vi "Example_OE1311&OE1351 Trig in.vi"() -> ()   [LabVIEW 2011]
panel:
  in  "Parameter Index":u16(ring) items=["X", "Y", "R", "θ", "XD1", "YD1", "RD1", "θD1", "XD2", "YD2", "RD2", "θD2", "XD3", "YD3", "RD3", "θD3", "XD4", "YD4", "RD4", "θD4", "XD5", "YD5", "RD5", "θD5", "XD6", "YD6", "RD6", "θD6", "XD7", "YD7", "RD7", "θD7", "X_Noise", "Y_Noise", "Frequency", "AUX-IN1", "AUX-IN2"]
  in  "Trig Mode":u8(ring) items=["Ext_Rissing_Edge", "Ext_Falling_Edge", "Ext_Bilateral_Edge", "Ext_High_Level", "Ext_Low_Level"]
  in  "Trig Source":u8(ring) items=["Internal", "Aux-in1", "Aux-in2"]
  out "Wave":dbl(graph)
  out "loss count":i32=-1
  out "Group":u32
  out "Error out":errorcluster caption="error out"
  in  "function":T1(ring)
  in  "Connect":bool
  in  "Port":u32=10001
  in  "Timeout":u32=100
  in  "IP Address":string="192.168.1.1"
  in  "选项卡控件":enum32{"选项卡 "}(tab)
  in  "Sweep Mode":u16(ring) items=["Linear", "Log"]
  in  "Start Frequency(Hz)":dbl=1000.0 min=1e-05 max=60000000.0 format="%#.3f"
  in  "Stop Frequency(Hz)":dbl=5000.0 min=1e-05 max=60000000.0 format="%#.3f"
  in  "Linear Step Frequency(Hz)":dbl=1000.0 min=1e-05 max=60000000.0 format="%#.3f"
  in  "Log Step Percent(%)":dbl=10.0 min=-100.0 max=100.0 format="%#.2f"
  in  "Step Time(ms)":i32=1000 min=50 max=100000
  in  "Sweep Run Mode":u16(ring) items=["Stop", "Singal", "Loop"]
  in  "Interval Count":u32=1 min=1 max=100000
  in  "Ref_Source":u8(ring) items=["External", "Internal"]
  in  "Sweep":u16(ring) items=["OFF", "ON"]
  out "data_buffer":dbl[][](array[numeric])
  out "cnt":u16
  # "Tel          :   +86-020-84133345\nWebsite  :   www.ssi-instrument.com\nE-mail     :   support@si-instrument.com"
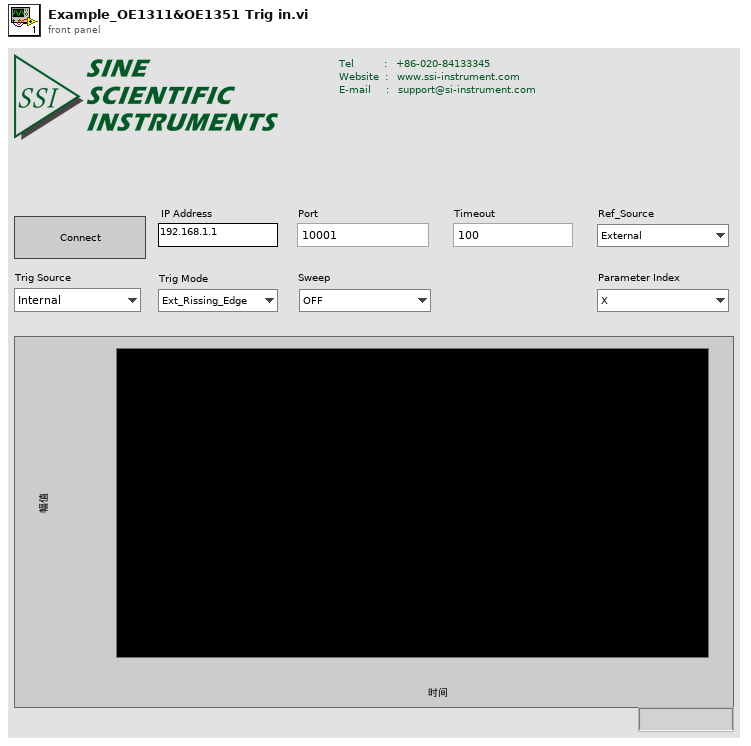
[diagram p1: front panel]
types:
  T1 = enum16{"initial", "Trig In Type", "Sample", "Ext_Sweep_Trig In", "Int_Sweep_Trig In"}
  T2 = enum8{"Enabled", "Disabled", "Disabled and Grayed Out"}
  T3 = cluster{"Port":u32, "Timeout":u32, "IP Address":string}
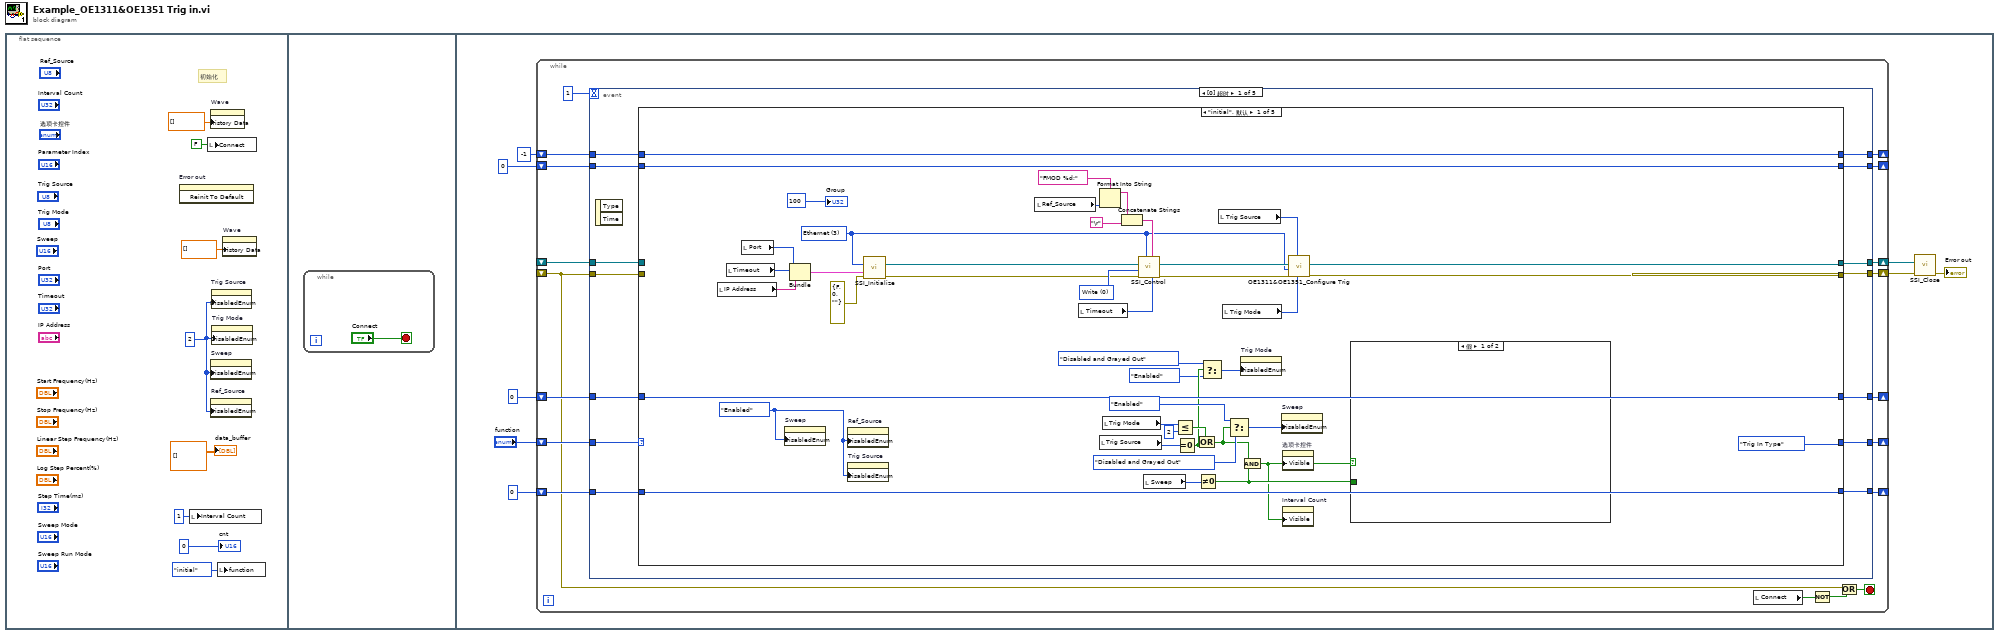
[diagram p0: block diagram]
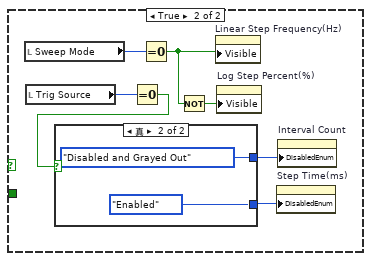
[diagram p2: hidden frame]
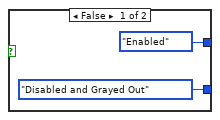
[diagram p3: hidden frame]
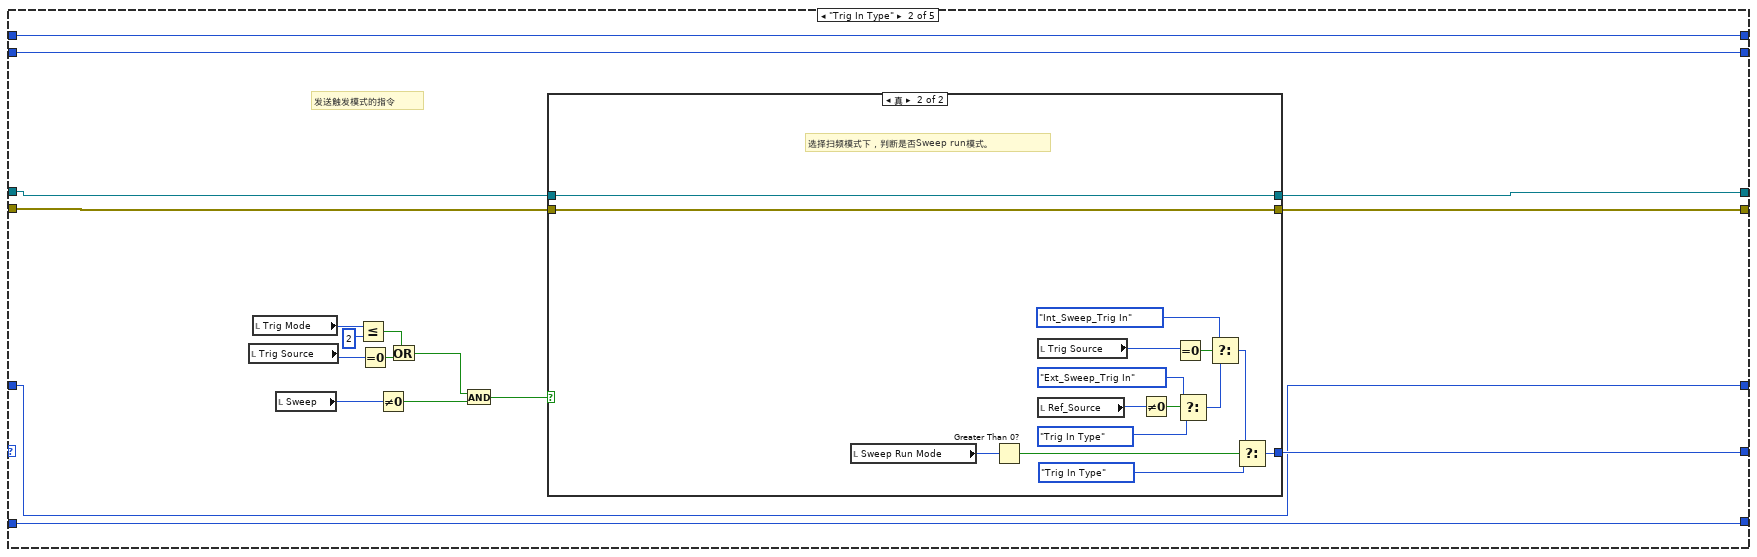
[diagram p4: hidden frame]
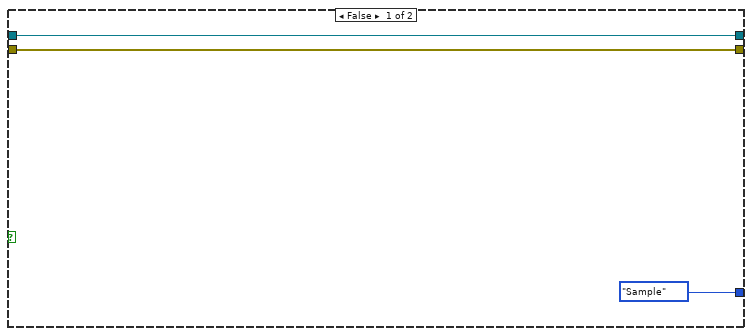
[diagram p5: hidden frame]
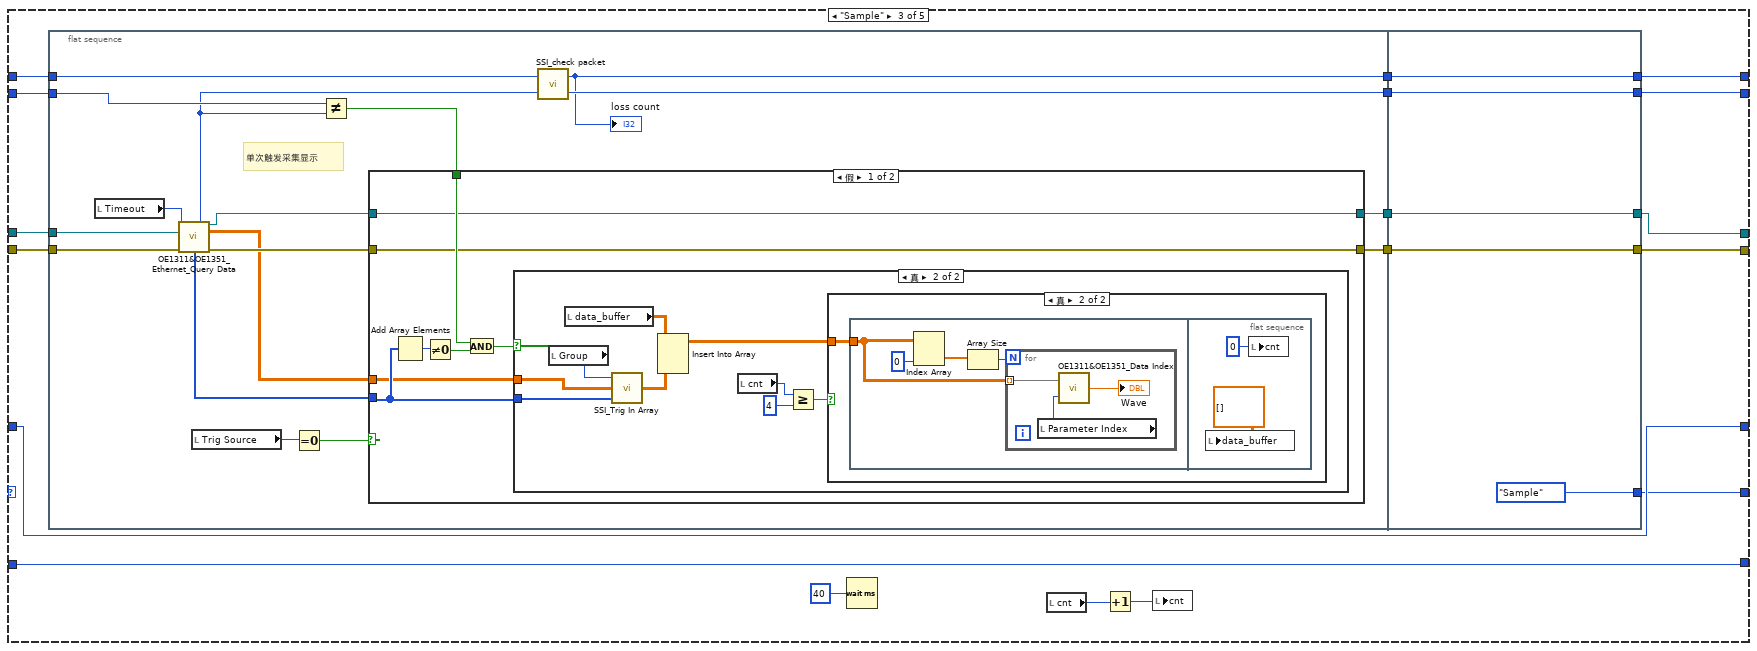
[diagram p6: hidden frame]
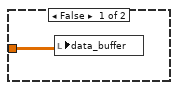
[diagram p8: hidden frame]
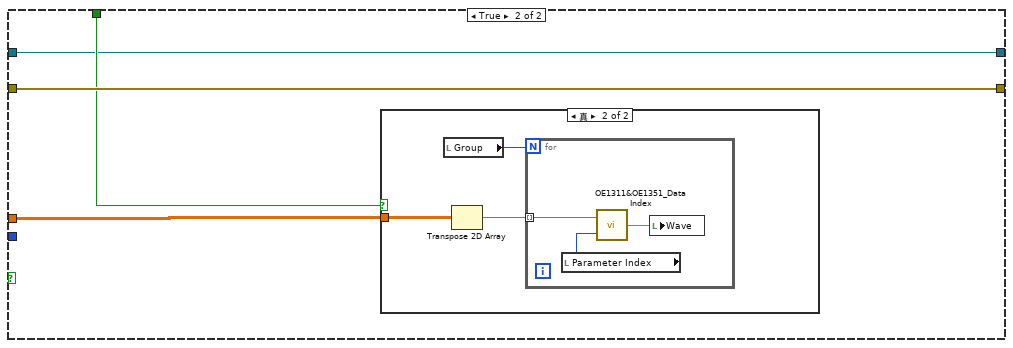
[diagram p9: hidden frame]
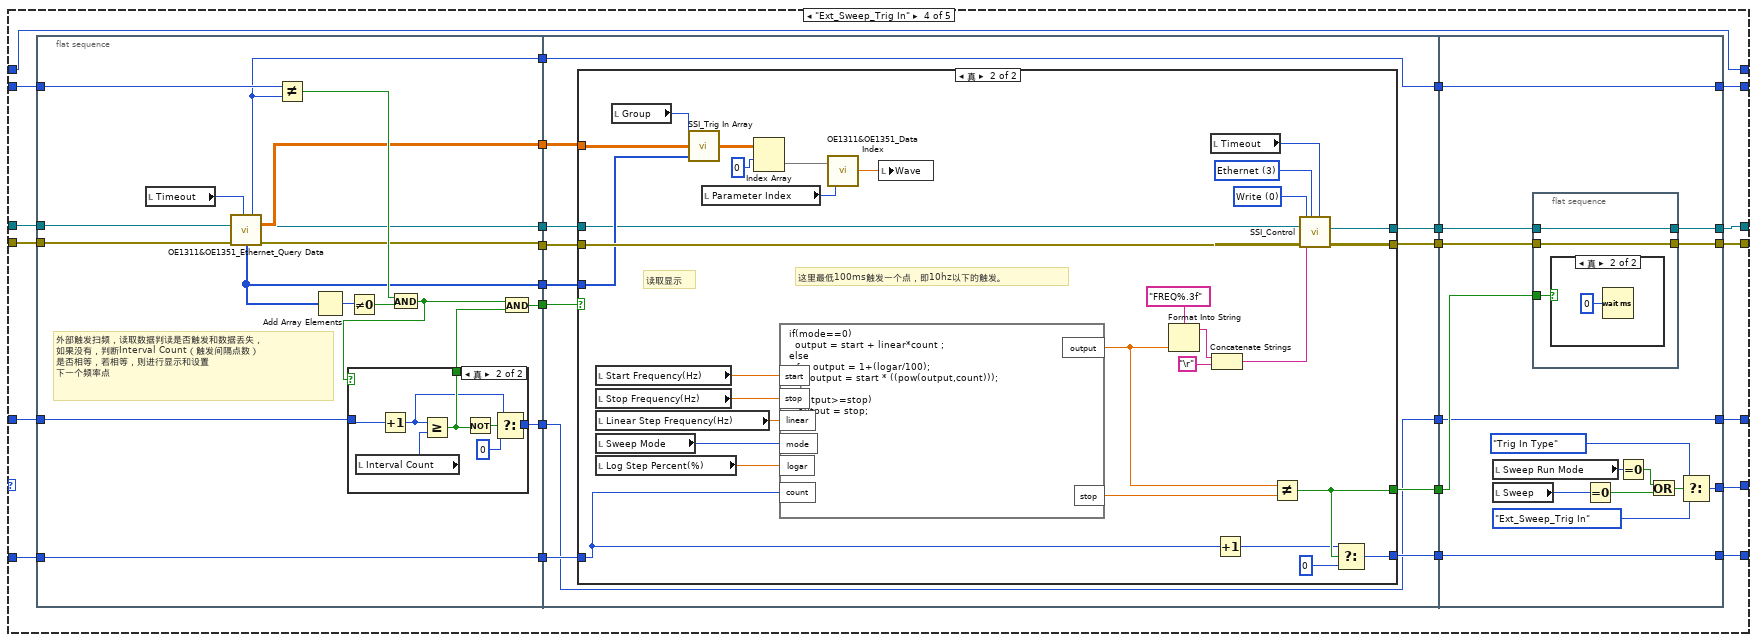
[diagram p11: hidden frame]
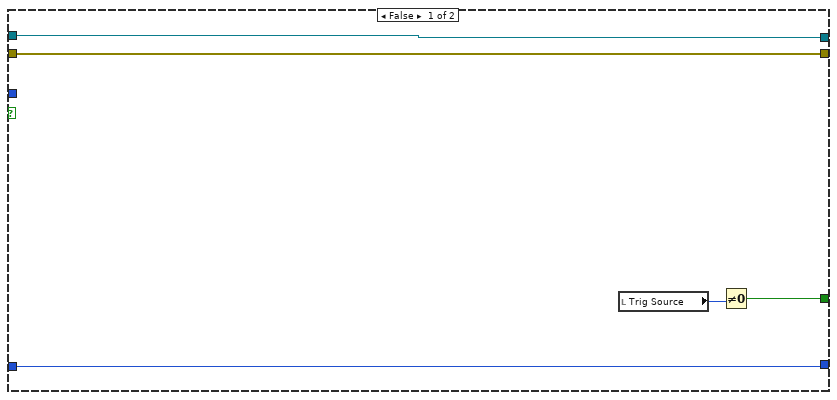
[diagram p13: hidden frame]
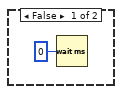
[diagram p14: hidden frame]
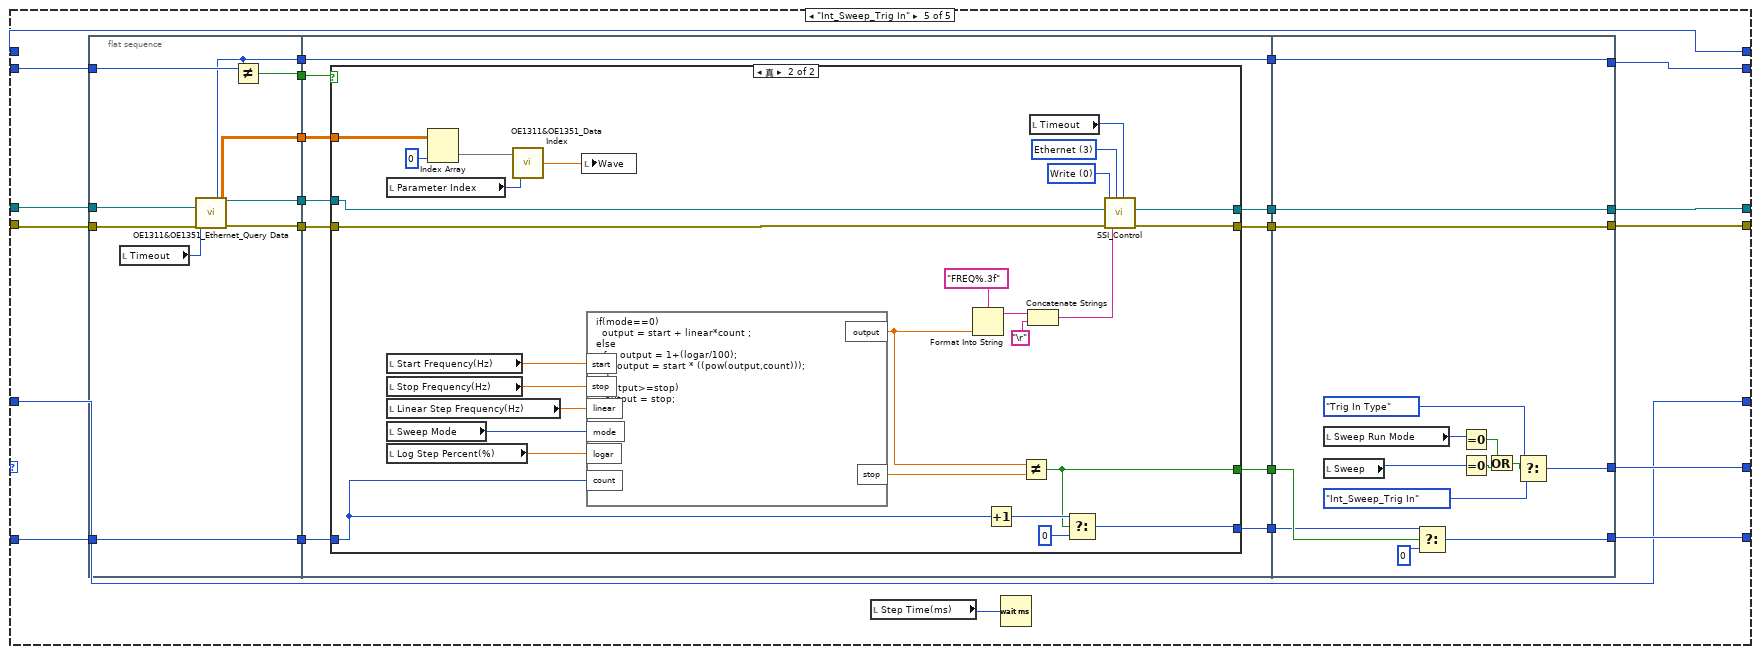
[diagram p15: hidden frame]
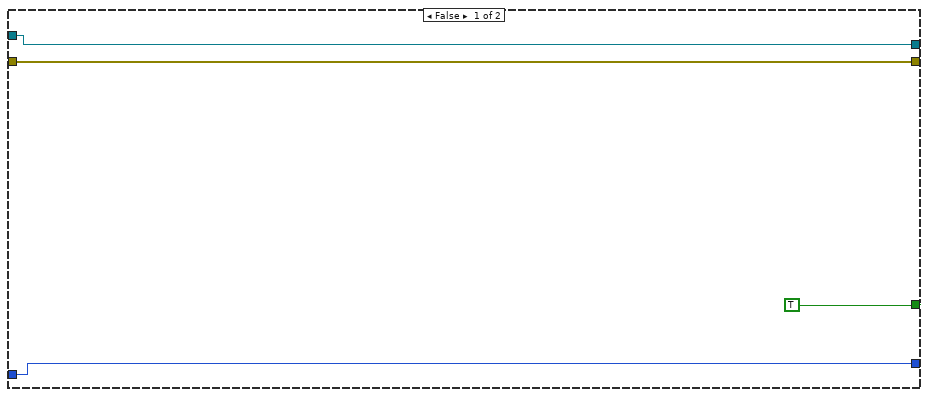
[diagram p16: hidden frame]
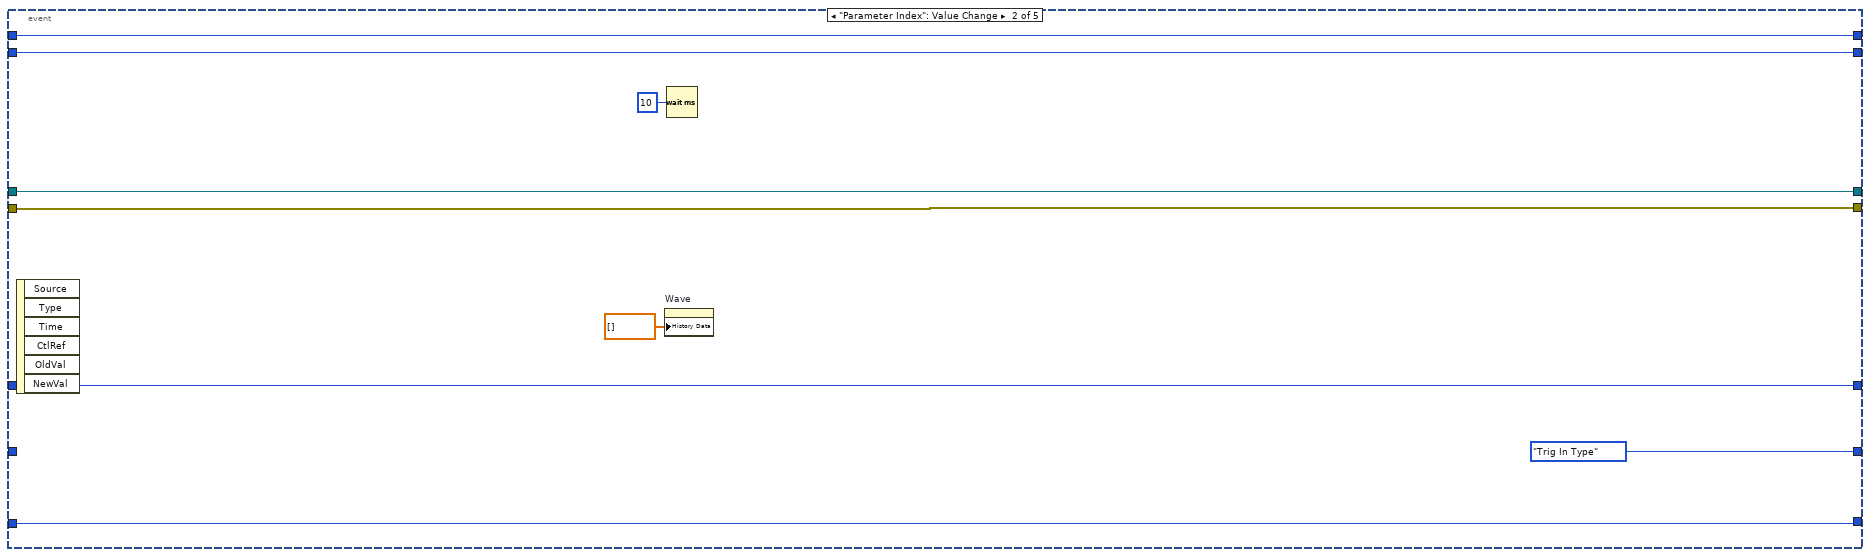
[diagram p17: hidden frame]
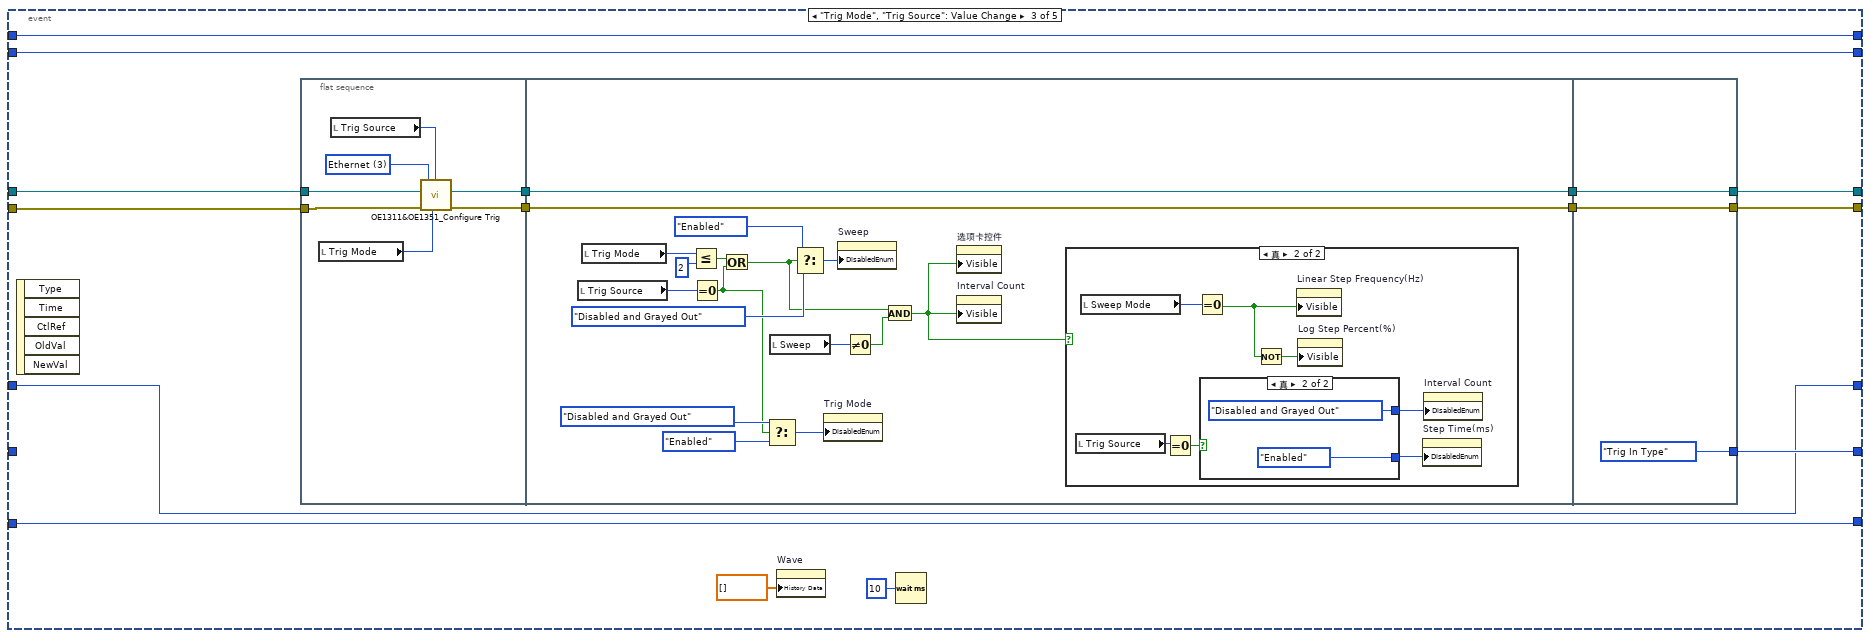
[diagram p18: hidden frame]
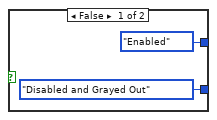
[diagram p20: hidden frame]
diagram:
  n1 = flat-sequence {
    frame #0 {
      w1 = 2
      # "初始化"
      n2 = invoke on="Error out" class="Clust (严格)" method="Reinit To Default"() -> ()  [unwired: 3 in, 3 out]
      n3 = local write "Interval Count"(u32 1 ("Interval Count")) -> ()
      n4 = local write "Connect"(FALSE ("Connect")) -> ()
      n5 = property on="Wave" class="WFChart (严格)"("History Data"=dbl[] [] ("历史数据")) -> ()  [unwired: 2 in, 2 out]
      n6 = property on="Sweep" class="Ring (严格)"("DisabledEnum"=w1) -> ()  [unwired: 2 in, 2 out]
      n7 = property on="Ref_Source" class="Ring (严格)"("DisabledEnum"=w1) -> ()  [unwired: 2 in, 2 out]
      n8 = property on="Trig Source" class="Ring (严格)"("DisabledEnum"=w1) -> ()  [unwired: 2 in, 2 out]
      n9 = property on="Trig Mode" class="Ring (严格)"("DisabledEnum"=w1) -> ()  [unwired: 2 in, 2 out]
      n10 = local write "function"(T1."initial" ("function")) -> ()
      n11 = property on="Wave" class="WFChart (严格)"("History Data"=dbl[] [] ("历史数据")) -> ()  [unwired: 2 in, 2 out]
      "data_buffer" <- dbl[][] []
      "cnt" <- 0
    }
    frame #1 {
      n12 = while {
        stop <- "Connect" stop-if-true
      }
    }
    frame #2 {
      n13 = while {
        shift-right: [w31] -> _
        shift-left: "function" -> [w32]
        shift-right: [w29] -> _
        shift-left: 0 ("f") -> [w30]
        shift-right: [w26] -> _
        shift-left: 0 -> [w27]
        shift-right: [w23] -> _
        shift-left: 0 -> [w24]
        shift-right: [w33] -> w16
        shift-left: _ -> [w22]
        shift-right: [w21] -> w12
        shift-left: _ -> [w20]
        shift-right: [w18] -> _
        shift-left: -1 ("loss count") -> [w19]
        stop <- w34 stop-if-true
        n14 = event shown="[0] 超时" {
          selector: _ -> [_ _ _ _ _]
          dyn-events: _ -> [_ _ _ _ _]
          timeout: 1 -> [_ _ _ _ _]
          tunnel: [w49 w434 w440 w497 w514] -> w33
          tunnel: w22 -> [w48 w434 w444 w498 w514]
          tunnel: w32 -> [w47 _ _ w501 _]
          tunnel: [w46 T1."Trig In Type" ("function") w446 w501 T1."Trig In Type" ("function")] -> w31
          tunnel: w30 -> [w45 w436 w451 w502 w510]
          tunnel: [w44 w436 w451 w502 w510] -> w29
          tunnel: w27 -> [w43 w432 w450 w499 w512]
          tunnel: [w42 w432 w450 w499 w512] -> w26
          tunnel: w24 -> [w41 w431 w445 w500 w509]
          tunnel: [w40 w431 w445 w500 w509] -> w23
          tunnel: [w39 w429 w437 w495 w513] -> w21
          tunnel: w20 -> [w38 w429 w443 w496 w513]
          tunnel: w19 -> [w37 w428 w447 w491 w511]
          tunnel: [w36 w428 w447 w491 w511] -> w18
          event Timeout {
            n15 = event-data() -> ()  [unwired: 1 in, 2 out]
            n16 = case shown="\"initial\", 默认" w47 {
              tunnel: w48 -> [_ w121 w156 w242 w348]
              tunnel: [w81 w120 w149 w240 w358] -> w49
              tunnel: [T1."Trig In Type" ("function") w119 w154 w231 w356] -> w46
              tunnel: w45 -> [w91 w118 w157 w241 w357]
              tunnel: [w91 w118 w157 w239 w355] -> w44
              tunnel: w43 -> [w89 w117 w153 w238 w360]
              tunnel: [w89 w117 w151 w237 w359] -> w42
              tunnel: w41 -> [w90 w116 w155 w225 w354]
              tunnel: [w90 w116 w155 w222 w354] -> w40
              tunnel: [w82 w111 w142 w219 w340] -> w39
              tunnel: w38 -> [_ w112 w144 w221 w344]
              tunnel: w37 -> [w73 w110 w147 w218 w339]
              tunnel: [w73 w110 w141 w218 w339] -> w36
              frame "initial", Default {
                w52 = u16 3 items=["USB", "RS232", "GPIB", "Ethernet"] ("Remote Mode")
                w70 = T2."Enabled" ("禁用")
                w75 = u16 0 items=["Write", "Read"] ("Control")
                n17 = local read "IP Address"() -> (w78:string)
                n18 = local read "Timeout"() -> (w79:u32)
                n19 = local read "Port"() -> (w80:u32)
                n20 = property on="Sweep" class="Ring (严格)"("DisabledEnum"=w70) -> ()  [unwired: 2 in, 2 out]
                n21 = Bundle("Port"=w80, "Timeout"=w79, "IP Address"=w78) -> (w77:T3)  [unwired: 1 in]
                n22 = property on="Ref_Source" class="Ring (严格)"("DisabledEnum"=w70) -> ()  [unwired: 2 in, 2 out]
                n23 = property on="Trig Source" class="Ring (严格)"("DisabledEnum"=w70) -> ()  [unwired: 2 in, 2 out]
                n24 = call "SSI_Initialize.vi"("Remote Mode"=w52, "Ethernet"=w77, "error in (no error)"=errorcluster {"status"=FALSE, "code"=0, "source"=""}) -> ("connection ID(Ethernet)"=w51:refnum<k5>, "error out"=w50:errorcluster)  [unwired: 10 in, 1 out]
                n25 = local read "Ref_Source"() -> (w87:u8)
                n26 = local read "Timeout"() -> (w71:u32)
                n27 = Format Into String(format string="FMOD %d;" ("格式字符串"), w87) -> (resulting string=w88:string)  [unwired: 2 in, 1 out]
                n28 = local read "Trig Source"() -> (w60:u8)
                n29 = local read "Trig Mode"() -> (w58:u8)
                n30 = Concatenate Strings(w88, "\r") -> (w74:string)
                n31 = call "SSI_Control.vi"("Tineout"=w71, "Write Buffer"=w74, "Remote Mode"=w52, "Error in (no error)"=w50, "Control"=w75, "Connection ID in"=w51) -> ("Error out"=w83:errorcluster, "Connection ID out"=w84:refnum<k5>)  [unwired: 2 in, 2 out]
                n32 = local read "Sweep"() -> (w64:u16)
                n33 = Less Or Equal?(x=w58, y=u8 2) -> (x <= y?=w59:bool)
                n34 = Equal To 0?(x=w60) -> (x = 0?=w56:bool)
                n35 = Or(x=w59, y=w56) -> (x .or. y?=w57:bool)
                n36 = Not Equal To 0?(x=w64) -> (x != 0?=w67:bool)
                n37 = Select(t=T2."Disabled and Grayed Out" ("禁用"), s=w56, f=T2."Enabled" ("禁用")) -> (s? t:f=w55:T2)
                n38 = local read "Trig Source"() -> (w68:u8)
                n39 = local read "Trig Mode"() -> (w69:u8)
                n40 = Select(t=T2."Enabled" ("禁用"), s=w57, f=T2."Disabled and Grayed Out") -> (s? t:f=w62:T2)
                n41 = property on="Trig Mode" class="Ring (严格)"("DisabledEnum"=w55) -> ()  [unwired: 2 in, 2 out]
                n42 = And(x=w57, y=w67) -> (x .and. y?=w66:bool)
                n43 = property on="Sweep" class="Ring (严格)"("DisabledEnum"=w62) -> ()  [unwired: 2 in, 2 out]
                n44 = property on="选项卡控件" class="TabCtl (严格)"("Visible"=w66) -> ()  [unwired: 2 in, 2 out]
                n45 = property on="Interval Count" class="DigNum (严格)"("Visible"=w66) -> ()  [unwired: 2 in, 2 out]
                n46 = call "OE1311&OE1351_Configure Trig.vi"("Trig Mode"=w69, "Trig Source"=w68, "Error in (no error)"=w83, "Remote Mode"=w52, "Connection ID in"=w84) -> ("Error out"=w81:errorcluster, "Connection ID out"=w82:refnum<k5>)  [unwired: 3 in, 2 out]
                n47 = case shown="假" w66 {
                  tunnel: w67 -> [_ _]
                  frame False {
                  }
                  frame True {
                    n48 = local read "Sweep Mode"() -> (w98:u16)
                    n49 = local read "Trig Source"() -> (w93:u8)
                    n50 = Equal To 0?(x=w93) -> (x = 0?=w94:bool)
                    n51 = case shown="真" w94 {
                      tunnel: [T2."Disabled and Grayed Out" ("禁用") T2."Enabled" ("禁用")] -> w96
                      tunnel: [T2."Enabled" ("禁用") T2."Disabled and Grayed Out" ("禁用")] -> w95
                      frame False {
                      }
                      frame True {
                      }
                    }
                    n52 = Equal To 0?(x=w98) -> (x = 0?=w99:bool)
                    n53 = Not(x=w99) -> (.not. x?=w97:bool)
                    n54 = property on="Linear Step Frequency(Hz)" class="DigNum (严格)"("Visible"=w99) -> ()  [unwired: 2 in, 2 out]
                    n55 = property on="Log Step Percent(%)" class="DigNum (严格)"("Visible"=w97) -> ()  [unwired: 2 in, 2 out]
                    n56 = property on="Step Time(ms)" class="DigNum (严格)"("DisabledEnum"=w96) -> ()  [unwired: 2 in, 2 out]
                    n57 = property on="Interval Count" class="DigNum (严格)"("DisabledEnum"=w95) -> ()  [unwired: 2 in, 2 out]
                  }
                }
                "Group" <- 100
              }
              frame "Trig In Type" {
                # "发送触发模式的指令"
                n58 = local read "Trig Source"() -> (w106:u8)
                n59 = local read "Trig Mode"() -> (w109:u8)
                n60 = local read "Sweep"() -> (w114:u16)
                n61 = Less Or Equal?(x=w109, y=u8 2) -> (x <= y?=w107:bool)
                n62 = Equal To 0?(x=w106) -> (x = 0?=w108:bool)
                n63 = Not Equal To 0?(x=w114) -> (x != 0?=w113:bool)
                n64 = Or(x=w107, y=w108) -> (x .or. y?=w104:bool)
                n65 = And(x=w104, y=w113) -> (x .and. y?=w115:bool)
                n66 = case shown="真" w115 {
                  tunnel: [w124 w135] -> w120
                  tunnel: w121 -> [w124 w135]
                  tunnel: [T1."Sample" ("function") w138] -> w119
                  tunnel: w112 -> [w122 w126]
                  tunnel: [w122 w126] -> w111
                  frame False {
                  }
                  frame True {
                    # "选择扫频模式下，判断是否Sweep run模式。"
                    n67 = local read "Sweep Run Mode"() -> (w136:u16)
                    n68 = Greater Than 0?(x=w136) -> (x > 0?=w139:bool)
                    n69 = local read "Trig Source"() -> (w125:u8)
                    n70 = local read "Ref_Source"() -> (w134:u8)
                    n71 = Not Equal To 0?(x=w134) -> (x != 0?=w133:bool)
                    n72 = Equal To 0?(x=w125) -> (x = 0?=w131:bool)
                    n73 = Select(t=T1."Ext_Sweep_Trig In" ("function"), s=w133, f=T1."Trig In Type" ("function")) -> (s? t:f=w132:T1)
                    n74 = Select(t=T1."Int_Sweep_Trig In" ("function"), s=w131, f=w132) -> (s? t:f=w137:T1)
                    n75 = Select(t=w137, s=w139, f=T1."Trig In Type" ("function")) -> (s? t:f=w138:T1)
                  }
                }
              }
              frame "Sample" {
                n76 = flat-sequence {
                  tunnel: w156 -> [w173]
                  tunnel: w153 -> [w170]
                  tunnel: [w167] -> w152
                  tunnel: [w168] -> w150
                  tunnel: w147 -> [w166]
                  tunnel: w144 -> [w164]
                  tunnel: [w162] -> w143
                  tunnel: [w161] -> w140
                  tunnel: w152 -> [w216]
                  tunnel: w150 -> [w215]
                  tunnel: [T1."Sample" ("function")] -> w154
                  tunnel: [w216] -> w151
                  tunnel: [w215] -> w149
                  tunnel: w143 -> [w213]
                  tunnel: [w213] -> w142
                  tunnel: [w212] -> w141
                  tunnel: w140 -> [w212]
                  frame #0 {
                    # "单次触发采集显示"
                    n77 = local read "Timeout"() -> (w160:u32)
                    n78 = call "OE1311&OE1351_Ethernet_Query Data.vi"("Connection ID in"=w164, "Timeout"=w160, "Error in (no error)"=w173) -> ("Buffer Count"=w167:u8, "Connection ID out"=w163:refnum<k5>, "Total Date Array"=w165:dbl[][], "Trig_Count"=w171:u8[], "Error out"=w169:errorcluster)  [unwired: 5 in, 3 out]
                    n79 = local read "Trig Source"() -> (w159:u8)
                    n80 = Equal To 0?(x=w159) -> (x = 0?=w172:bool)
                    n81 = Not Equal?(x=w170, y=w167) -> (x != y?=w158:bool)
                    n82 = case shown="假" w172 {
                      tunnel: w165 -> [w177 w204]
                      tunnel: w171 -> [w180 _]
                      tunnel: w158 -> [w176 w203]
                      tunnel: w169 -> [w174 w205]
                      tunnel: [w174 w205] -> w168
                      tunnel: w163 -> [w175 w202]
                      tunnel: [w175 w202] -> w162
                      frame False {
                        n83 = Add Array Elements(numeric array=w180) -> (sum=w181:u8)
                        n84 = Not Equal To 0?(x=w181) -> (x != 0?=w179:bool)
                        n85 = And(x=w176, y=w179) -> (x .and. y?=w178:bool)
                        n86 = case shown="真" w178 {
                          tunnel: w177 -> [_ w190]
                          tunnel: w180 -> [_ w189]
                          frame False {
                          }
                          frame True {
                            n87 = local read "Group"() -> (w188:u32)
                            n88 = local read "data_buffer"() -> (w187:dbl[][])
                            n89 = call "SSI_Trig In Array.vi"("Trig_Count"=w189, "Input Array"=w190, "Group"=w188) -> ("Output Array"=w186:dbl[][])
                            n90 = Insert Into Array(array=w187, new element=w186) -> (w185:dbl[][])  [unwired: 2 in]
                            n91 = local read "cnt"() -> (w184:u16)
                            n92 = Greater Or Equal?(x=w184, y=u16 4) -> (x >= y?=w182:bool)
                            n93 = case shown="真" w182 {
                              tunnel: w185 -> [w191 w192]
                              frame False {
                                n94 = local write "data_buffer"(w191) -> ()
                              }
                              frame True {
                                n95 = flat-sequence {
                                tunnel: w192 -> [w194]
                                frame #0 {
                                n96 = Index Array(array=w194, index (col)=0 ("禁用的索引 (列)")) -> (element=w193:dbl[])  [unwired: 1 in]
                                n97 = Array Size(array=w193) -> (size(s)=w196:i32)
                                n98 = for {
                                N: w196 -> [_]
                                tunnel: w194 -> [w198] mode=indexing
                                n99 = local read "Parameter Index"() -> (w197:u16)
                                n100 = call "OE1311&OE1351_Data Index.vi"("Parameter Type"=w197, "Input Date Array"=w198) -> ("Parameter"=→"Wave":dbl)
                                }
                                }
                                frame #1 {
                                n101 = local write "data_buffer"(dbl[][] [] ("data_buffer")) -> ()
                                n102 = local write "cnt"(u16 0 ("cnt")) -> ()
                                }
                                }
                              }
                            }
                          }
                        }
                      }
                      frame True {
                        n103 = case shown="真" w203 {
                          tunnel: w204 -> [_ w208]
                          frame False {
                          }
                          frame True {
                            n104 = local read "Group"() -> (w207:u32)
                            n105 = Transpose 2D Array(2D array=w208) -> (transposed array=w206:dbl[][])
                            n106 = for {
                              N: w207 -> [_]
                              tunnel: w206 -> [w211] mode=indexing
                              n107 = local read "Parameter Index"() -> (w209:u16)
                              n108 = call "OE1311&OE1351_Data Index.vi"("Parameter Type"=w209, "Input Date Array"=w211) -> ("Parameter"=w210:dbl)
                              n109 = local write "Wave"(w210) -> ()
                            }
                          }
                        }
                      }
                    }
                    n110 = call "SSI_check packet.vi"("input"=w167, "input loss"=w166) -> ("loss count"=w161:i32)  [unwired: 1 out]
                    "loss count" <- w161
                  }
                  frame #1 {
                  }
                }
                n111 = Wait (ms)(milliseconds to wait=40) -> ()  [unwired: 1 out]
                n112 = local read "cnt"() -> (w145:u16)
                n113 = Increment(x=w145) -> (x+1=w146:u16)
                n114 = local write "cnt"(w146) -> ()
              }
              frame "Ext_Sweep_Trig In" {
                n115 = flat-sequence {
                  tunnel: w242 -> [w259]
                  tunnel: w241 -> [w257]
                  tunnel: w238 -> [w260]
                  tunnel: [w257] -> w236
                  tunnel: [w258] -> w235
                  tunnel: [w253] -> w229
                  tunnel: [w252] -> w228
                  tunnel: [w251] -> w227
                  tunnel: [w250] -> w226
                  tunnel: w225 -> [w248]
                  tunnel: [w246] -> w224
                  tunnel: w221 -> [w245]
                  tunnel: [w244] -> w217
                  tunnel: w235 -> [w271]
                  tunnel: w236 -> [w278]
                  tunnel: [w279] -> w234
                  tunnel: [w277] -> w233
                  tunnel: [w271] -> w232
                  tunnel: [w276] -> w230
                  tunnel: w229 -> [w280]
                  tunnel: w228 -> [w275]
                  tunnel: w227 -> [w274]
                  tunnel: w226 -> [w273]
                  tunnel: w224 -> [w272]
                  tunnel: [w272] -> w223
                  tunnel: [w270] -> w220
                  tunnel: w217 -> [w269]
                  tunnel: [w331] -> w237
                  tunnel: [w332] -> w239
                  tunnel: [w329] -> w240
                  tunnel: w234 -> [w330]
                  tunnel: w233 -> [w332]
                  tunnel: w232 -> [w331]
                  tunnel: [w326] -> w231
                  tunnel: w230 -> [w328]
                  tunnel: w223 -> [w327]
                  tunnel: [w327] -> w222
                  tunnel: w220 -> [w322]
                  tunnel: [w321] -> w219
                  frame #0 {
                    # "外部触发扫频，读取数据判读是否触发和数据丢失，\n如果没有，判断Interval Count（触发间隔点数）\n是否相等，若相等，则进行显示和设置\n下一个频率点"
                    n116 = local read "Timeout"() -> (w243:u32)
                    n117 = call "OE1311&OE1351_Ethernet_Query Data.vi"("Connection ID in"=w245, "Timeout"=w243, "Error in (no error)"=w259) -> ("Buffer Count"=w258:u8, "Connection ID out"=w244:refnum<k5>, "Total Date Array"=w252:dbl[][], "Trig_Count"=w251:u8[], "Error out"=w253:errorcluster)  [unwired: 5 in, 3 out]
                    n118 = Not Equal?(x=w260, y=w258) -> (x != y?=w255:bool)
                    n119 = Add Array Elements(numeric array=w251) -> (sum=w256:u8)
                    n120 = Not Equal To 0?(x=w256) -> (x != 0?=w254:bool)
                    n121 = And(x=w255, y=w254) -> (x .and. y?=w249:bool)
                    n122 = case shown="真" w249 {
                      tunnel: w248 -> [w261 w268]
                      tunnel: [_ w265] -> w247
                      tunnel: [w261 w262] -> w246
                      frame False {
                      }
                      frame True {
                        n123 = local read "Interval Count"() -> (w267:u32)
                        n124 = Increment(x=w268) -> (x+1=w264:i32)
                        n125 = Greater Or Equal?(x=w264, y=w267) -> (x >= y?=w265:bool)
                        n126 = Not(x=w265) -> (.not. x?=w266:bool)
                        n127 = Select(t=w264, s=w266, f=0) -> (s? t:f=w262:i32)
                      }
                    }
                    n128 = And(x=w249, y=w247) -> (x .and. y?=w250:bool)
                  }
                  frame #1 {
                    n129 = case shown="真" w273 {
                      tunnel: w280 -> [w285 w299]
                      tunnel: [w285 w301] -> w279
                      tunnel: w278 -> [w284 w307]
                      tunnel: [w284 w306] -> w277
                      tunnel: [w283 w305] -> w276
                      tunnel: w275 -> [_ w298]
                      tunnel: w274 -> [_ w296]
                      tunnel: w269 -> [w282 w293]
                      tunnel: [w282 w292] -> w270
                      frame False {
                        n130 = local read "Trig Source"() -> (w281:u8)
                        n131 = Not Equal To 0?(x=w281) -> (x != 0?=w283:bool)
                      }
                      frame True {
                        w289 = u16 3 items=["USB", "RS232", "GPIB", "Ethernet"] ("Remote Mode")
                        w291 = u16 0 items=["Write", "Read"] ("Control")
                        # "这里最低100ms触发一个点，即10hz以下的触发。"
                        # "读取显示"
                        n132 = local read "Start Frequency(Hz)"() -> (w313:dbl)
                        n133 = local read "Stop Frequency(Hz)"() -> (w312:dbl)
                        n134 = local read "Linear Step Frequency(Hz)"() -> (w311:dbl)
                        n135 = local read "Sweep Mode"() -> (w310:u16)
                        n136 = local read "Log Step Percent(%)"() -> (w309:dbl)
                        n137 = local read "Group"() -> (w297:u32)
                        n138 = call "SSI_Trig In Array.vi"("Trig_Count"=w296, "Input Array"=w298, "Group"=w297) -> ("Output Array"=w295:dbl[][])
                        n139 = local read "Parameter Index"() -> (w288:u16)
                        n140 = Index Array(array=w295, index (row)=0 ("索引 (行)")) -> (element=w294:dbl[])  [unwired: 1 in]
                        n141 = formula code="if(mode==0)\n  output = start + linear*count ;\nelse \n  {    output = 1+(logar/100);\n       output = start * ((pow(output,count)));\n   }\nif(output>=stop)\n   output = stop;"("start"=w313, "stop"=w312, "linear"=w311, "logar"=w309, "mode"=w310, "count"=w307) -> ("stop"=w308:dbl, "output"=w302:dbl)
                        n142 = call "OE1311&OE1351_Data Index.vi"("Parameter Type"=w288, "Input Date Array"=w294) -> ("Parameter"=w287:dbl)
                        n143 = local write "Wave"(w287) -> ()
                        n144 = Format Into String(format string="FREQ%.3f" ("格式字符串"), w302) -> (resulting string=w315:string)  [unwired: 2 in, 1 out]
                        n145 = local read "Timeout"() -> (w290:u32)
                        n146 = Concatenate Strings(w315, "\r") -> (w300:string)
                        n147 = Increment(x=w307) -> (x+1=w304:i32)
                        n148 = Not Equal?(x=w302, y=w308) -> (x != y?=w305:bool)
                        n149 = call "SSI_Control.vi"("Tineout"=w290, "Write Buffer"=w300, "Remote Mode"=w289, "Error in (no error)"=w299, "Control"=w291, "Connection ID in"=w293) -> ("Error out"=w301:errorcluster, "Connection ID out"=w292:refnum<k5>)  [unwired: 2 in, 2 out]
                        n150 = Select(t=w304, s=w305, f=0) -> (s? t:f=w306:i32)
                      }
                    }
                  }
                  frame #2 {
                    n151 = local read "Sweep Run Mode"() -> (w317:u16)
                    n152 = local read "Sweep"() -> (w325:u16)
                    n153 = flat-sequence {
                      tunnel: [w335] -> w329
                      tunnel: w330 -> [w335]
                      tunnel: w328 -> [w334]
                      tunnel: [w333] -> w321
                      tunnel: w322 -> [w333]
                      frame #0 {
                        n154 = case shown="真" w334 {
                          frame False {
                            n155 = Wait (ms)(milliseconds to wait=u32 0 ("等待时间（毫秒）")) -> ()  [unwired: 1 out]
                          }
                          frame True {
                            n156 = Wait (ms)(milliseconds to wait=u32 0 ("等待时间（毫秒）")) -> ()  [unwired: 1 out]
                          }
                        }
                      }
                    }
                    n157 = Equal To 0?(x=w325) -> (x = 0?=w319:bool)
                    n158 = Equal To 0?(x=w317) -> (x = 0?=w318:bool)
                    n159 = Or(x=w318, y=w319) -> (x .or. y?=w320:bool)
                    n160 = Select(t=T1."Trig In Type" ("function"), s=w320, f=T1."Ext_Sweep_Trig In" ("function")) -> (s? t:f=w326:T1)
                  }
                }
              }
              frame "Int_Sweep_Trig In" {
                n161 = flat-sequence {
                  tunnel: [w367] -> w353
                  tunnel: [w366] -> w351
                  tunnel: w360 -> [w370]
                  tunnel: w357 -> [w368]
                  tunnel: w348 -> [w365]
                  tunnel: [w369] -> w347
                  tunnel: [w368] -> w346
                  tunnel: w344 -> [w364]
                  tunnel: [w363] -> w343
                  tunnel: [w362] -> w342
                  tunnel: w353 -> [w380]
                  tunnel: [w380] -> w352
                  tunnel: w351 -> [w379]
                  tunnel: [w378] -> w350
                  tunnel: [w374] -> w349
                  tunnel: w347 -> [w377]
                  tunnel: w346 -> [w376]
                  tunnel: [w375] -> w345
                  tunnel: w343 -> [w373]
                  tunnel: w342 -> [w372]
                  tunnel: [w371] -> w341
                  tunnel: [w427] -> w359
                  tunnel: w352 -> [w427]
                  tunnel: [w426] -> w358
                  tunnel: w350 -> [w426]
                  tunnel: [w420] -> w356
                  tunnel: [w425] -> w355
                  tunnel: w349 -> [w423]
                  tunnel: w345 -> [w422]
                  tunnel: w341 -> [w417]
                  tunnel: [w417] -> w340
                  frame #0 {
                    n162 = local read "Timeout"() -> (w361:u32)
                    n163 = call "OE1311&OE1351_Ethernet_Query Data.vi"("Connection ID in"=w364, "Timeout"=w361, "Error in (no error)"=w365) -> ("Buffer Count"=w367:u8, "Connection ID out"=w362:refnum<k5>, "Total Date Array"=w363:dbl[][], "Error out"=w366:errorcluster)  [unwired: 5 in, 4 out]
                    n164 = Not Equal?(x=w370, y=w367) -> (x != y?=w369:bool)
                  }
                  frame #1 {
                    n165 = case shown="真" w377 {
                      tunnel: [w384 w394] -> w378
                      tunnel: w379 -> [w384 w395]
                      tunnel: w376 -> [w383 w406]
                      tunnel: [w383 w400] -> w375
                      tunnel: [TRUE w401] -> w374
                      tunnel: w373 -> [_ w392]
                      tunnel: w372 -> [w381 w391]
                      tunnel: [w381 w389] -> w371
                      frame False {
                      }
                      frame True {
                        w387 = u16 3 items=["USB", "RS232", "GPIB", "Ethernet"] ("Remote Mode")
                        w390 = u16 0 items=["Write", "Read"] ("Control")
                        n166 = local read "Parameter Index"() -> (w386:u16)
                        n167 = local read "Start Frequency(Hz)"() -> (w412:dbl)
                        n168 = local read "Stop Frequency(Hz)"() -> (w411:dbl)
                        n169 = local read "Linear Step Frequency(Hz)"() -> (w410:dbl)
                        n170 = local read "Sweep Mode"() -> (w409:u16)
                        n171 = local read "Log Step Percent(%)"() -> (w408:dbl)
                        n172 = Index Array(array=w392, index (col)=0 ("禁用的索引 (列)")) -> (element=w396:dbl[])  [unwired: 1 in]
                        n173 = call "OE1311&OE1351_Data Index.vi"("Parameter Type"=w386, "Input Date Array"=w396) -> ("Parameter"=w385:dbl)
                        n174 = local write "Wave"(w385) -> ()
                        n175 = formula code="if(mode==0)\n  output = start + linear*count ;\nelse \n  {    output = 1+(logar/100);\n       output = start * ((pow(output,count)));\n   }\nif(output>=stop)\n   output = stop;"("start"=w412, "stop"=w411, "linear"=w410, "logar"=w408, "mode"=w409, "count"=w406) -> ("stop"=w402:dbl, "output"=w398:dbl)
                        n176 = Format Into String(format string="FREQ%.3f" ("格式字符串"), w398) -> (resulting string=w403:string)  [unwired: 2 in, 1 out]
                        n177 = Increment(x=w406) -> (x+1=w407:i32)
                        n178 = Not Equal?(x=w398, y=w402) -> (x != y?=w401:bool)
                        n179 = Concatenate Strings(w403, "\r") -> (w393:string)
                        n180 = local read "Timeout"() -> (w388:u32)
                        n181 = Select(t=w407, s=w401, f=0) -> (s? t:f=w400:i32)
                        n182 = call "SSI_Control.vi"("Tineout"=w388, "Write Buffer"=w393, "Remote Mode"=w387, "Error in (no error)"=w395, "Control"=w390, "Connection ID in"=w391) -> ("Error out"=w394:errorcluster, "Connection ID out"=w389:refnum<k5>)  [unwired: 2 in, 2 out]
                      }
                    }
                  }
                  frame #2 {
                    n183 = local read "Sweep Run Mode"() -> (w413:u16)
                    n184 = local read "Sweep"() -> (w421:u16)
                    n185 = Select(t=w422, s=w423, f=u16 0) -> (s? t:f=w425:i32)
                    n186 = Equal To 0?(x=w413) -> (x = 0?=w414:bool)
                    n187 = Equal To 0?(x=w421) -> (x = 0?=w415:bool)
                    n188 = Or(x=w414, y=w415) -> (x .or. y?=w416:bool)
                    n189 = Select(t=T1."Trig In Type" ("function"), s=w416, f=T1."Int_Sweep_Trig In" ("function")) -> (s? t:f=w420:T1)
                  }
                }
                n190 = local read "Step Time(ms)"() -> (w338:i32)
                n191 = Wait (ms)(milliseconds to wait=w338) -> ()  [unwired: 1 out]
              }
            }
          }
          event "Parameter Index": Value Change {
            n192 = event-data() -> ()  [unwired: 1 in, 6 out]
            n193 = property on="Wave" class="WFChart (严格)"("History Data"=dbl[] [] ("历史数据")) -> ()  [unwired: 2 in, 2 out]
            n194 = Wait (ms)(milliseconds to wait=u32 10 ("等待时间（毫秒）")) -> ()  [unwired: 1 out]
          }
          event "Trig Mode", "Trig Source": Value Change {
            n195 = event-data() -> ()  [unwired: 1 in, 5 out]
            n196 = flat-sequence {
              tunnel: w444 -> [w457]
              tunnel: w443 -> [w458]
              tunnel: [w455] -> w441
              tunnel: [w454] -> w438
              tunnel: [w468] -> w442
              tunnel: w441 -> [w468]
              tunnel: [w467] -> w439
              tunnel: w438 -> [w467]
              tunnel: [T1."Trig In Type" ("function")] -> w446
              tunnel: w442 -> [w488]
              tunnel: [w488] -> w440
              tunnel: w439 -> [w487]
              tunnel: [w487] -> w437
              frame #0 {
                w456 = u16 3 items=["USB"=0, "Ethernet"=3] ("Remote Mode")
                n197 = local read "Trig Mode"() -> (w453:u8)
                n198 = local read "Trig Source"() -> (w452:u8)
                n199 = call "OE1311&OE1351_Configure Trig.vi"("Trig Mode"=w453, "Trig Source"=w452, "Error in (no error)"=w457, "Remote Mode"=w456, "Connection ID in"=w458) -> ("Error out"=w455:errorcluster, "Connection ID out"=w454:refnum<k5>)  [unwired: 3 in, 2 out]
              }
              frame #1 {
                n200 = local read "Trig Source"() -> (w464:u8)
                n201 = local read "Trig Mode"() -> (w463:u8)
                n202 = Less Or Equal?(x=w463, y=u8 2) -> (x <= y?=w466:bool)
                n203 = Equal To 0?(x=w464) -> (x = 0?=w459:bool)
                n204 = Or(x=w466, y=w459) -> (x .or. y?=w465:bool)
                n205 = Select(t=T2."Disabled and Grayed Out" ("禁用"), s=w459, f=T2."Enabled" ("禁用")) -> (s? t:f=w462:T2)
                n206 = local read "Sweep"() -> (w470:u16)
                n207 = Select(t=T2."Enabled" ("禁用"), s=w465, f=T2."Disabled and Grayed Out") -> (s? t:f=w474:T2)
                n208 = property on="Trig Mode" class="Ring (严格)"("DisabledEnum"=w462) -> ()  [unwired: 2 in, 2 out]
                n209 = property on="Sweep" class="Ring (严格)"("DisabledEnum"=w474) -> ()  [unwired: 2 in, 2 out]
                n210 = Not Equal To 0?(x=w470) -> (x != 0?=w469:bool)
                n211 = And(x=w465, y=w469) -> (x .and. y?=w471:bool)
                n212 = property on="选项卡控件" class="TabCtl (严格)"("Visible"=w471) -> ()  [unwired: 2 in, 2 out]
                n213 = property on="Interval Count" class="DigNum (严格)"("Visible"=w471) -> ()  [unwired: 2 in, 2 out]
                n214 = case shown="真" w471 {
                  frame False {
                  }
                  frame True {
                    n215 = local read "Trig Source"() -> (w476:u8)
                    n216 = local read "Sweep Mode"() -> (w481:u16)
                    n217 = Equal To 0?(x=w476) -> (x = 0?=w477:bool)
                    n218 = Equal To 0?(x=w481) -> (x = 0?=w482:bool)
                    n219 = case shown="真" w477 {
                      tunnel: [T2."Disabled and Grayed Out" ("禁用") T2."Enabled" ("禁用")] -> w479
                      tunnel: [T2."Enabled" ("禁用") T2."Disabled and Grayed Out" ("禁用")] -> w478
                      frame False {
                      }
                      frame True {
                      }
                    }
                    n220 = Not(x=w482) -> (.not. x?=w480:bool)
                    n221 = property on="Linear Step Frequency(Hz)" class="DigNum (严格)"("Visible"=w482) -> ()  [unwired: 2 in, 2 out]
                    n222 = property on="Log Step Percent(%)" class="DigNum (严格)"("Visible"=w480) -> ()  [unwired: 2 in, 2 out]
                    n223 = property on="Step Time(ms)" class="DigNum (严格)"("DisabledEnum"=w479) -> ()  [unwired: 2 in, 2 out]
                    n224 = property on="Interval Count" class="DigNum (严格)"("DisabledEnum"=w478) -> ()  [unwired: 2 in, 2 out]
                  }
                }
              }
              frame #2 {
              }
            }
            n225 = property on="Wave" class="WFChart (严格)"("History Data"=dbl[] [] ("历史数据")) -> ()  [unwired: 2 in, 2 out]
            n226 = Wait (ms)(milliseconds to wait=u32 10 ("等待时间（毫秒）")) -> ()  [unwired: 1 out]
          }
          event "Ref_Source": Value Change {
            w490 = u16 3 items=["USB", "RS232", "GPIB", "Ethernet"] ("Remote Mode")
            w506 = u16 0 items=["Write", "Read"] ("Control")
            n227 = event-data() -> ()  [unwired: 1 in, 5 out]
            n228 = local read "Ref_Source"() -> (w504:u8)
            n229 = Format Into String(format string="FMOD %d;" ("格式字符串"), w504) -> (resulting string=w503:string)  [unwired: 2 in, 1 out]
            n230 = Concatenate Strings(w503, "\r") -> (w507:string)
            n231 = call "SSI_Control.vi"("Write Buffer"=w507, "Remote Mode"=w490, "Error in (no error)"=w498, "Control"=w506, "Connection ID in"=w496) -> ("Error out"=w497:errorcluster, "Connection ID out"=w495:refnum<k5>)  [unwired: 3 in, 2 out]
            n232 = Wait (ms)(milliseconds to wait=u32 10 ("等待时间（毫秒）")) -> ()  [unwired: 1 out]
            n233 = property on="Wave" class="WFChart (严格)"("History Data"=dbl[] [] ("历史数据")) -> ()  [unwired: 2 in, 2 out]
          }
          event "Sweep": Value Change {
            n234 = event-data() -> ()  [unwired: 1 in, 5 out]
            n235 = local read "Sweep"() -> (w516:u16)
            n236 = Not Equal To 0?(x=w516) -> (x != 0?=w508:bool)
            n237 = property on="选项卡控件" class="TabCtl (严格)"("Visible"=w508) -> ()  [unwired: 2 in, 2 out]
            n238 = property on="Interval Count" class="DigNum (严格)"("Visible"=w508) -> ()  [unwired: 2 in, 2 out]
            n239 = case shown="真" w508 {
              frame False {
              }
              frame True {
                n240 = local read "Trig Mode"() -> (w518:u8)
                n241 = local read "Sweep Mode"() -> (w523:u16)
                n242 = Equal To 0?(x=w518) -> (x = 0?=w519:bool)
                n243 = Equal To 0?(x=w523) -> (x = 0?=w524:bool)
                n244 = case shown="假" w519 {
                  tunnel: [T2."Disabled and Grayed Out" ("禁用") T2."Enabled" ("禁用")] -> w521
                  tunnel: [T2."Enabled" ("禁用") T2."Disabled and Grayed Out" ("禁用")] -> w520
                  frame False {
                  }
                  frame True {
                  }
                }
                n245 = Not(x=w524) -> (.not. x?=w522:bool)
                n246 = property on="Linear Step Frequency(Hz)" class="DigNum (严格)"("Visible"=w524) -> ()  [unwired: 2 in, 2 out]
                n247 = property on="Log Step Percent(%)" class="DigNum (严格)"("Visible"=w522) -> ()  [unwired: 2 in, 2 out]
                n248 = property on="Step Time(ms)" class="DigNum (严格)"("DisabledEnum"=w521) -> ()  [unwired: 2 in, 2 out]
                n249 = property on="Interval Count" class="DigNum (严格)"("DisabledEnum"=w520) -> ()  [unwired: 2 in, 2 out]
              }
            }
            n250 = property on="Wave" class="WFChart (严格)"("History Data"=dbl[] [] ("历史数据")) -> ()  [unwired: 2 in, 2 out]
          }
        }
        n251 = local read "Connect"() -> (w25:bool)
        n252 = Not(x=w25) -> (.not. x?=w35:bool)
        n253 = Or(x=w22, y=w35) -> (x .or. y?=w34:bool)
      }
      n254 = call "SSI_Close.vi"("Error in (no error)"=w16, "Connection ID in"=w12) -> ("Error out"=→"Error out":errorcluster)  [unwired: 5 in]
    }
  }
